vi "Read Connection Ref.vi"(8 "error in (no error)":errorcluster, 11 "MySQL in":refnum<class "MySQL.lvclass">) -> (0 "error out":errorcluster, 2 "connection reference":T1, 3 "MySQL out":refnum<class "MySQL.lvclass">)   [LabVIEW 2021, in "Database.lvlib" / "MySQL.lvclass"]
uses:
  MySQL.lvclass
  <vilib>/addons/database/Connection.llb/Conn ObjectReference.ctl
  DB/DB.lvclass
  <vilib>/addons/database/NI_Database_API.lvlib
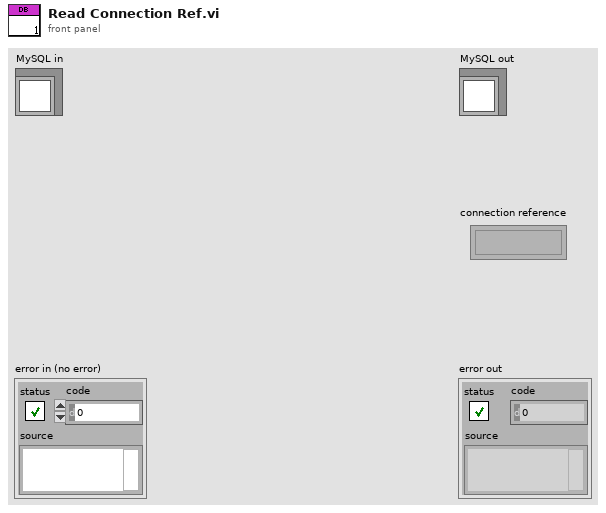
[diagram p1: front panel]
types:
  T1 = typedef "NI_Database_API.lvlib/Conn ObjectReference.ctl" = refnum<k1>
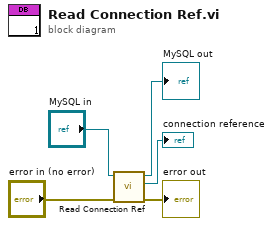
[diagram p0: block diagram]
diagram:
  n1 = call-parent "Read Connection Ref.vi"("error in (no error)"="error in (no error)", "DB in"="MySQL in") -> ("error out"=→"error out":errorcluster, "connection reference"=→"connection reference":T1, "DB out"=→"MySQL out":refnum<class "MySQL.lvclass">)  [unwired: 7 in]
